vi "LAStop.vi"(8 "Error In":errorcluster, 10 "TaskId":string, 11 "LiteAgent In":T1) -> (0 "Error Out":errorcluster, 3 "LiteAgent Out":T1)   [LabVIEW 2017, in "LiteAgentSDK.lvlib"]
uses:
  LiteAgentSDK.lvlib
  C:/Users/Jan/Projects/LiteAgentSDK-LabVIEW/Source/Bin/LiteAgentSDK.LabVIEW.dll
  Bin/LiteAgentSDK.LabVIEW.dll
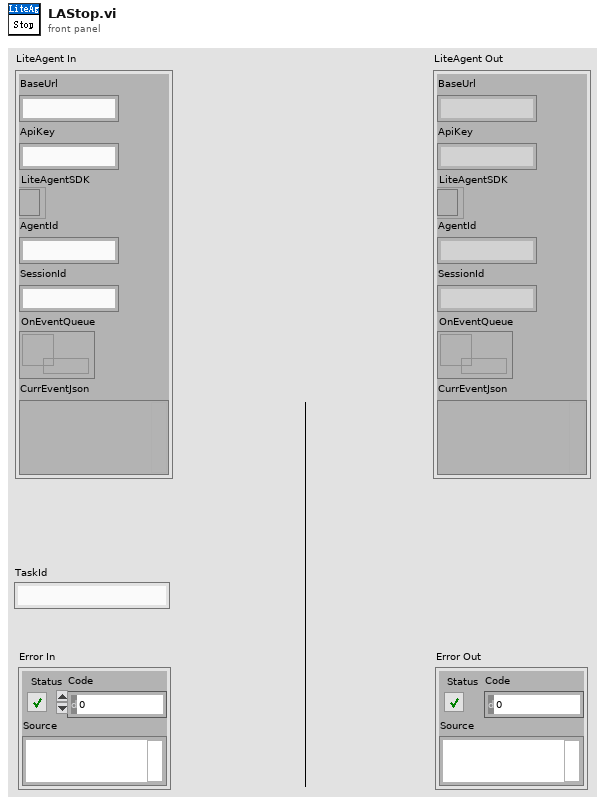
[diagram p1: front panel]
types:
  T1 = cluster{"BaseUrl":string, "ApiKey":string, "LiteAgentSDK":refnum<k24>, "AgentId":string, "SessionId":string, "OnEventQueue":refnum<queue>, "CurrEventJson":variant}
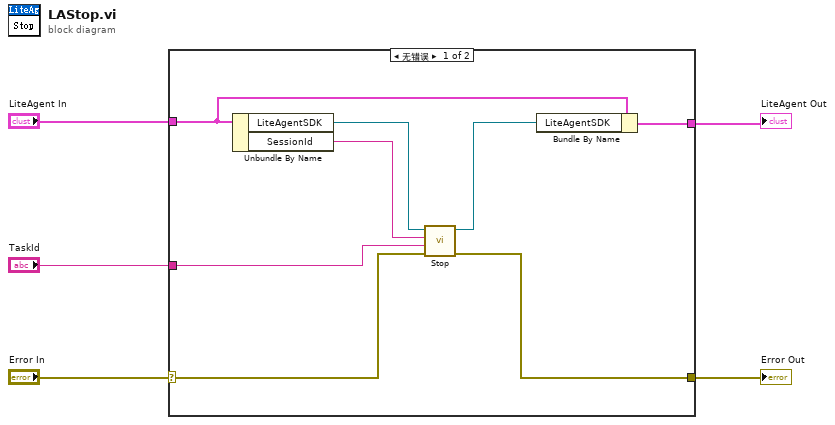
[diagram p0: block diagram]
diagram:
  n1 = case shown="无错误" "Error In" {
    selector: "Error In" -> [w11 w15]
    tunnel: [w10 w15] -> w4
    tunnel: "TaskId" -> [w7 _]
    tunnel: "LiteAgent In" -> [w13 w14]
    tunnel: [w12 w14] -> w1
    frame No Error {
      n2 = Unbundle By Name(w13) -> ("LiteAgentSDK"=w9:refnum<k24>, "SessionId"=w6:string)
      n3 = call "Stop.vi"("Error Input"=w11, "TaskId"=w7, "SessionId"=w6, "LiteAgentSDK Input"=w9) -> ("Error Output"=w10:errorcluster, "LiteAgentSDK Output"=w8:refnum<k24>)  [unwired: 6 in]
      n4 = Bundle By Name(cluster=w13, "LiteAgentSDK"=w8) -> (w12:T1)
    }
    frame Error {
    }
  }
  "Error Out" <- w4
  "LiteAgent Out" <- w1
